vi "RSZVB Get Frequency Conversion Type.vi"(8 "error in (no error)":errorcluster {"code" format="%.0x"}, 11 "VISA session":refnum<visa-resource-name>) -> (0 "error out":errorcluster {"code" format="%.0x"}, 2 "Converter Type":string, 3 "dup VISA session":refnum<visa-resource-name>)   [LabVIEW 2011]
doc: "This VI returns the frequency converter type for enhanced frequency-converting measurements (with option ZVA-K8, Enhanced Frequency Conversion). \n\nNote(s):\n\n(1) This VI is available only on R&S ZVA and ZVT instrument.\n\nRemote-control command(s):\nSENSe<Ch>:FREQuency:CONVersion:DEVice:NAME?"
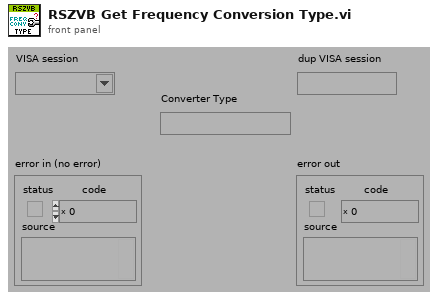
[diagram p1: front panel]
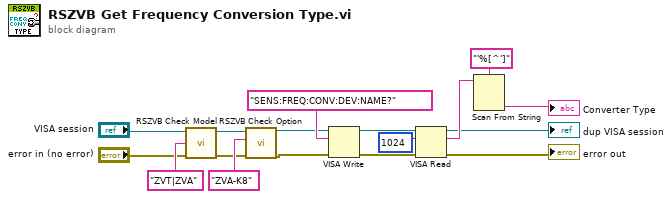
[diagram p0: block diagram]
diagram:
  n1 = call "RSZVB Check Model.vi"("error in (no error)"="error in (no error)", "Model"="ZVT|ZVA" ("Options"), "VISA session"="VISA session") -> ("error out"=w8:errorcluster, "dup VISA session"=w9:refnum<visa-resource-name>)  [unwired: 7 in]
  n2 = call "RSZVB Check Option.vi"("error in (no error)"=w8, "Options"="ZVA-K8", "VISA session"=w9) -> ("error out"=w7:errorcluster, "dup VISA session"=w6:refnum<visa-resource-name>)  [unwired: 7 in]
  n3 = VISA Write(VISA resource name=w6, write buffer="SENS:FREQ:CONV:DEV:NAME?", error in (no error)=w7) -> (VISA resource name out=w16:refnum<visa-resource-name>, error out=w15:errorcluster)  [unwired: 1 out]
  n4 = VISA Read(VISA resource name=w16, byte count=u32 1024 ("byte count (0)"), error in (no error)=w15) -> (VISA resource name out=→"dup VISA session":refnum<visa-resource-name>, read buffer=w12:string, error out=→"error out":errorcluster)  [unwired: 1 out]
  n5 = Scan From String(format string="'%[^']", input string=w12) -> (output 1=→"Converter Type":string)  [unwired: 3 in, 3 out]
